vi "Get Properties.vi"(8 "error in (no error)":errorcluster, 11 "App Properties in":refnum<class "App Properties.lvclass">) -> (0 "error out":errorcluster, 2 "Class Properties":T1 {"Mode" items=["Operator"=0, "Engineering"=1, "Verification"=6]}, 3 "App Properties out":refnum<class "App Properties.lvclass">)   [LabVIEW 2017, in "Application.lvlib" / "App Properties.lvclass"]
uses:
  App Properties.lvclass
  Class/typedefs/Test Info -- Cluster.ctl
  Class/Application.lvclass
  Class Properties -- Cluster.ctl
  Golden Board/Class/Golden Board.lvclass
  Test Recipe/Class/Test Recipe.lvclass
  UUT Reference -- Cluster.ctl
  Class/typedefs/Op Mode -- Enum.ctl
  Station Config/Class/Station Config.lvclass
  Instruments/Instrument/Class/Instrument.lvclass
  Test Result -- Cluster.ctl
  <vilib>/TSS/ACRObat Test Framework/Classes/Variable Engine/Class/Variable Engine.lvclass
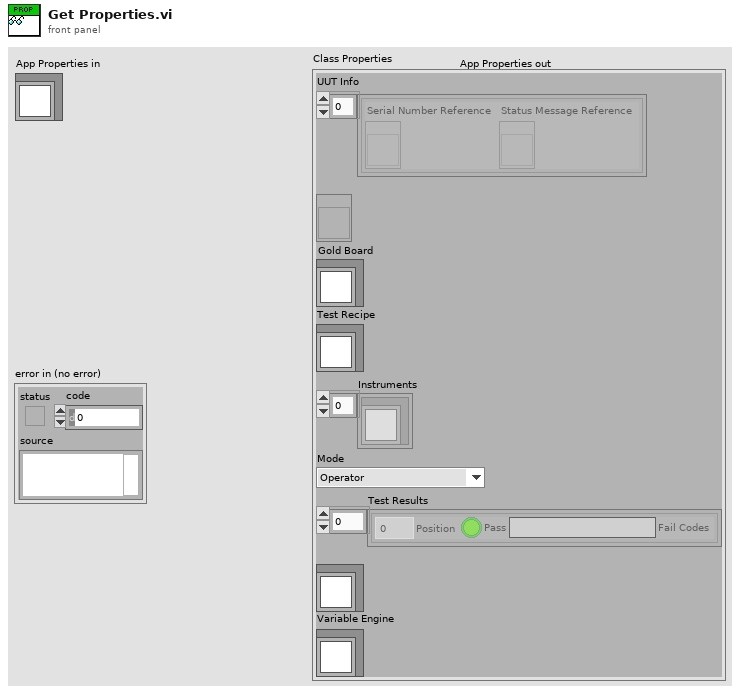
[diagram p1: front panel]
types:
  T1 = typedef "Application.lvlib/App Properties.lvclass/Class Properties -- Cluster.ctl" = cluster{"UUT Info":T2[], "Test Information":refnum<vi>, "Gold Board":refnum<class "Golden Board.lvclass">, "Test Recipe":refnum<class "Test Recipe.lvclass">, "Instruments":refnum<class "Instrument.lvclass">[], "Mode":T3, "Test Results":T4[], "Station Config":refnum<class "Station Config.lvclass">, "Variable Engine":refnum<class "Variable Engine.lvclass">}
  T2 = typedef "Application.lvlib/App Properties.lvclass/UUT Reference -- Cluster.ctl" = cluster{"Serial Number Reference":refnum<vi>, "Status Message Reference":refnum<vi>}
  T3 = typedef "Application.lvlib/Application.lvclass/Op Mode -- Enum.ctl" = u16
  T4 = typedef "Application.lvlib/App Properties.lvclass/Test Result -- Cluster.ctl" = cluster{"Position":i32, "Pass":bool, "Fail Codes":string}
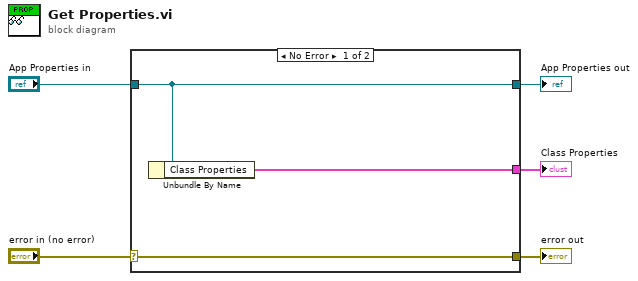
[diagram p0: block diagram]
diagram:
  n1 = case shown="No Error" "error in (no error)" {
    selector: "error in (no error)" -> [w8 w9]
    tunnel: [w8 w9] -> w4
    tunnel: [w7 w10] -> w2
    tunnel: "App Properties in" -> [w7 w10]
    tunnel: [w6 _] -> w1
    frame No Error {
      n2 = Unbundle By Name(w7) -> ("Class Properties"=w6:T1)
    }
    frame Error {
    }
  }
  "error out" <- w4
  "App Properties out" <- w2
  "Class Properties" <- w1
